vi "ContourPlot v2_no_I.vi"() -> ()   [LabVIEW 2024]
uses:
  <vilib>/Utility/file.llb/Read Delimited Spreadsheet (DBL).vi
  <vilib>/Analysis/NI_AALBase.lvlib
  <vilib>/gmath/NI_Gmath.lvlib
panel:
  out "Ready?":bool=TRUE
  in  "Auto x axis T":bool
  in  "Tab Control 2":enum32{"Contour", "Curve"}(tab)
  out "Intensity Graph":dbl[][](graph)
  out "XY Graph":cluster{"Y":dbl[], "Y":dbl[]}[](graph)=[{"Y"=[0.0, 0.1, 0.2, 0.3, 0.4, 0.5, 0.6, 0.7, 0.8, 0.9, 1.0, 1.1, 1.2, 1.3, 1.4, 1.5, 1.6, 1.7, 1.8, 1.9, 2.0, 2.1, 2.2, 2.3, 2.4, 2.5, 2.6, 2.7, 2.8, 2.9, 3.0, 3.1, 3.2, 3.3, 3.4, 3.5, 3.6, 3.7, 3.8, 3.9, 4.0, 4.1, 4.2, 4.3, 4.4, 4.5, 4.6, 4.7, 4.8, 4.9, 5.0, 4.9, 4.8, 4.7, 4.6, 4.5, 4.4, 4.3, 4.2, 4.1, 4.0, 3.9, 3.8, 3.7, 3.6, 3.5, 3.4, 3.3, 3.2, 3.1, 3.0, 2.9, 2.8, 2.7, 2.6, 2.5, 2.4, 2.3, 2.2, 2.1, 2.0, 1.9, 1.8, 1.7, 1.6, 1.5, 1.4, 1.3, 1.2, 1.1, 1.0, 0.9, 0.8, 0.7, 0.6, 0.5, 0.4, 0.3, 0.2, 0.1, 0.0, -0.1, -0.2, -0.3, -0.4, -0.5, -0.6, -0.7, -0.8, -0.9, -1.0, -1.1, -1.2, -1.3, -1.4, -1.5, -1.6, -1.7, -1.8, -1.9, -2.0, -2.1, -2.2, -2.3, -2.4, -2.5, -2.6, -2.7, -2.8, -2.9, -3.0, -3.1, -3.2, -3.3, -3.4, -3.5, -3.6, -3.7, -3.8, -3.9, -4.0, -4.1, -4.2, -4.3, -4.4, -4.5, -4.6, -4.7, -4.8, -4.9, -5.0, -4.9, -4.8, -4.7, -4.6, -4.5, -4.4, -4.3, -4.2, -4.1, -4.0, -3.9, -3.8, -3.7, -3.6, -3.5, -3.4, -3.3, -3.2, -3.1, -3.0, -2.9, -2.8, -2.7, -2.6, -2.5, -2.4, -2.3, -2.2, -2.1, -2.0, -1.9, -1.8, -1.7, -1.6, -1.5, -1.4, -1.3, -1.2, -1.1, -1.0, -0.9, -0.8, -0.7, -0.6, -0.5, -0.4, -0.3, -0.2, -0.1], "Y"=[-inf, -inf, -inf, -inf, -inf, -inf, -inf, -inf, -inf, -inf, -inf, -inf, -inf, -inf, -inf, -inf, -inf, -inf, 0.5607799884800001, 0.58669998848, 0.58669998848, 0.56749998848, 0.5578999884800001, 0.57805999616, 0.5502199961600001, 0.58285999424, -inf, -inf, -inf, -inf, -inf, 0.59917999424, 0.5905399884800001, 0.34573999616, 0.60301999616, 0.6529399884799999, 0.5290999884800001, 0.49549998848, 0.58669998848, 0.5953399884799999, 0.5876599884800001, 0.35149999616, 0.34478001152000004, 0.6097399884799999, 0.34765998848, 0.6250999884799999, 0.61933999424, 0.34478000576, 0.60493999616, 0.6030199884799999, 0.56653999424, 0.53389999424, 0.52717999616, 0.49645998848, 0.47725998848, 0.46477999711999995, 0.52429999424, 0.5358199884800001, 0.58957998848, 0.34478000576, 0.34765999424000005, 0.34478000576, -inf, -inf, 0.57805999424, 0.34478001152000004, -inf, -inf, 0.34573999616, -inf, -inf, -inf, -inf, -inf, -inf, -inf, -inf, -inf, -inf, -inf, -inf, -inf, -inf, -inf, -inf, -inf, -inf, -inf, -inf, -inf, -inf, -inf, -inf, -inf, -inf, -inf, -inf, -inf, -inf, -inf, -inf, -inf, -inf, -inf, -inf, -inf, -inf, -inf, -inf, -inf, -inf, -inf, -inf, -inf, -inf, -inf, -inf, -inf, -inf, -inf, -inf, -inf, 0.6519799884799999, -inf, -inf, 0.34765998848, 0.34669998848, -inf, 0.34478001152000004, 0.58957999424, 0.34573998848, 0.58957999616, 0.58957999424, 0.5550199884800001, 0.5886199884800001, 0.5617399884800001, 0.5905399884800001, 0.6519799884799999, 0.6202999942399999, 0.55309999424, 0.53005998848, 0.52045999424, 0.50509998848, 0.48109999423999994, 0.49741999616, 0.49453998847999997, 0.48301998848, 0.48301998848, 0.48109998847999996, 0.5310199884800001, 0.5905399884800001, 0.5905399884800001, 0.5262199884800001, 0.5646199884800001, 0.5905399884800001, 0.5751799884800001, 0.59629998848, 0.5818999980799999, 0.6164599884799999, 0.34478000576, -inf, -inf, -inf, -inf, -inf, 0.34573998848, -inf, -inf, 0.34478001152000004, -inf, 0.34478001152000004, -inf, -inf, -inf, -inf, -inf, -inf, -inf, -inf, -inf, -inf, -inf, -inf, -inf, -inf, -inf, -inf, -inf, -inf, -inf, -inf, -inf, 3.79790000576, 3.73550001152, -inf, -inf, -inf, -inf, -inf, -inf]}]
  in  "Voltage treshold":dbl=1.2e-05 format="%_3g"
  in  "Ignore points":i32=250
  in  "Tab Control":enum32{"Y cut ", "Y curve", "X cut"}(tab)=enum."Y curve"
  out "Y Cut":cluster{dbl[], "Intensity Graph":dbl[]}(graph)
  in  "intervals":i32=100
  out "Y Histogram":T1(graph)={"X Values"=[3.75038961, 3.75213283, 3.7538760499999997, 3.7556192699999995, 3.7573624899999993, 3.759105709999999, 3.760848929999999, 3.762592149999999, 3.7643353699999986, 3.7660785899999984, 3.7678218099999983, 3.769565029999998, 3.771308249999998, 3.7730514699999977, 3.7747946899999976, 3.7765379099999974, 3.778281129999997, 3.780024349999997, 3.781767569999997, 3.7835107899999967, 3.7852540099999965, 3.7869972299999963, 3.788740449999996, 3.790483669999996, 3.792226889999996, 3.7939701099999956, 3.7957133299999954, 3.7974565499999953, 3.799199769999995, 3.800942989999995, 3.8026862099999947, 3.8044294299999946, 3.8061726499999944, 3.807915869999994, 3.809659089999994, 3.811402309999994, 3.8131455299999937, 3.8148887499999935, 3.8166319699999933, 3.818375189999993, 3.820118409999993, 3.821861629999993, 3.8236048499999926, 3.8253480699999924, 3.8270912899999923, 3.828834509999992, 3.830577729999992, 3.8323209499999917, 3.8340641699999916, 3.8358073899999914, 3.837550609999991, 3.839293829999991, 3.841037049999991, 3.8427802699999907, 3.8445234899999905, 3.8462667099999903, 3.84800992999999, 3.84975314999999, 3.85149636999999, 3.8532395899999896, 3.8549828099999894, 3.8567260299999893, 3.858469249999989, 3.860212469999989, 3.8619556899999887, 3.8636989099999886, 3.8654421299999884, 3.867185349999988, 3.868928569999988, 3.870671789999988, 3.8724150099999877, 3.8741582299999875, 3.8759014499999873, 3.877644669999987, 3.879387889999987, 3.881131109999987, 3.8828743299999866, 3.8846175499999864, 3.8863607699999863, 3.888103989999986, 3.889847209999986, 3.8915904299999857, 3.8933336499999855, 3.8950768699999854, 3.896820089999985, 3.898563309999985, 3.900306529999985, 3.9020497499999847, 3.9037929699999845, 3.9055361899999843, 3.907279409999984, 3.909022629999984, 3.910765849999984, 3.9125090699999836, 3.9142522899999834, 3.9159955099999832, 3.917738729999983, 3.919481949999983, 3.9212251699999827, 3.9229683899999825], "Histogram: h(x)"=[1, 0, 0, 0, 0, 0, 0, 2, 0, 0, 0, 1, 0, 0, 1, 0, 1, 0, 0, 3, 2, 6, 5, 5, 4, 6, 5, 7, 5, 9, 11, 10, 7, 4, 13, 19, 20, 29, 21, 22, 20, 29, 41, 35, 44, 31, 43, 57, 50, 60, 68, 80, 88, 77, 95, 96, 111, 129, 153, 146, 164, 145, 201, 219, 230, 252, 254, 300, 343, 312, 361, 376, 335, 418, 424, 438, 448, 345, 399, 403, 331, 298, 293, 226, 209, 177, 126, 85, 86, 56, 28, 16, 15, 8, 2, 1, 1, 2, 0, 1]}
  in  "Histogram range":dbl=0.4
  out "X Cut":cluster{dbl[], "Intensity Graph":dbl[]}(graph)={[0.0, 0.1, 0.2, 0.30000000000000004, 0.4, 0.5, 0.6000000000000001, 0.7000000000000001, 0.8, 0.9, 1.0, 1.1, 1.2000000000000002, 1.3, 1.4000000000000001, 1.5, 1.6, 1.7000000000000002, 1.8, 1.9000000000000001, 2.0, 2.1, 2.2, 2.3000000000000003, 2.4000000000000004, 2.5, 2.6, 2.7, 2.8000000000000003, 2.9000000000000004, 3.0, 3.1, 3.2, 3.3000000000000003, 3.4000000000000004, 3.5, 3.6, 3.7, 3.8000000000000003, 3.9000000000000004, 4.0, 4.1000000000000005, 4.2, 4.3, 4.4, 4.5, 4.6000000000000005, 4.7, 4.800000000000001, 4.9, 5.0, 5.1000000000000005, 5.2, 5.300000000000001, 5.4, 5.5, 5.6000000000000005, 5.7, 5.800000000000001, 5.9, 6.0, 6.1000000000000005, 6.2, 6.300000000000001, 6.4, 6.5, 6.6000000000000005, 6.7, 6.800000000000001, 6.9, 7.0, 7.1000000000000005, 7.2, 7.300000000000001, 7.4, 7.5, 7.6000000000000005, 7.7, 7.800000000000001, 7.9, 8.0, 8.1, 8.200000000000001, 8.3, 8.4, 8.5, 8.6, 8.700000000000001, 8.8, 8.9, 9.0, 9.1, 9.200000000000001, 9.3, 9.4, 9.5, 9.600000000000001, 9.700000000000001, 9.8, 9.9, 10.0, 10.100000000000001, 10.200000000000001, 10.3, 10.4, 10.5, 10.600000000000001, 10.700000000000001, 10.8, 10.9, 11.0, 11.100000000000001, 11.200000000000001, 11.3, 11.4, 11.5, 11.600000000000001, 11.700000000000001, 11.8, 11.9, 12.0, 12.100000000000001, 12.200000000000001, 12.3, 12.4, 12.5, 12.600000000000001, 12.700000000000001, 12.8, 12.9, 13.0, 13.100000000000001, 13.200000000000001, 13.3, 13.4, 13.5, 13.600000000000001, 13.700000000000001, 13.8, 13.9, 14.0, 14.100000000000001, 14.200000000000001, 14.3, 14.4, 14.5, 14.600000000000001, 14.700000000000001, 14.8, 14.9, 15.0, 15.100000000000001, 15.200000000000001, 15.3, 15.4, 15.5, 15.600000000000001, 15.700000000000001, 15.8, 15.9, 16.0, 16.1, 16.2, 16.3, 16.400000000000002, 16.5, 16.6, 16.7, 16.8, 16.900000000000002, 17.0, 17.1, 17.2, 17.3, 17.400000000000002, 17.5, 17.6, 17.7, 17.8, 17.900000000000002, 18.0, 18.1, 18.2, 18.3, 18.400000000000002, 18.5, 18.6, 18.7, 18.8, 18.900000000000002, 19.0, 19.1, 19.200000000000003, 19.3, 19.400000000000002, 19.5, 19.6, 19.700000000000003, 19.8, 19.900000000000002], "Intensity Graph"=[0.0, 0.0, 0.0, 0.0, 0.0, 0.0, 4.0, 3.0, 0.0, 0.0, 0.0, 0.0, 0.0, 0.0, 0.0, 0.0, 0.0, 0.0, 0.0, 0.0, 0.0, 0.0, 0.0, 0.0, 0.0, 0.0, 0.0, 0.0, 0.0, 0.0, 0.0, 0.0, 0.0, 0.0, 0.0, 0.0, 0.0, 0.0, 0.0, 0.0, 0.0, 0.0, 0.0, 0.0, 0.0, 0.0, 0.0, 0.0, 0.0, 0.0, 0.0, 0.0, 0.0, 0.0, 0.0, 0.0, 0.0, 0.0, 0.0, 0.0, 0.0, 0.0, 0.0, 0.0, 0.0, 0.0, 0.0, 0.0, 0.0, 0.0, 0.0, 0.0, 0.0, 0.0, 0.0, 0.0, 0.0, 0.0, 0.0, 0.0, 0.0, 0.0, 0.0, 0.0, 0.0, 0.0, 0.0, 0.0, 0.0, 0.0, 0.0, 0.0, 0.0, 0.0, 0.0, 0.0, 0.0, 0.0, 0.0, 0.0, 0.0, 0.0, 0.0, 0.0, 0.0, 0.0, 114.0, 0.0, 0.0, 0.0, 0.0, 0.0, 0.0, 0.0, 0.0, 0.0, 0.0, 0.0, 0.0, 0.0, 0.0, 0.0, 0.0, 0.0, 0.0, 0.0, 0.0, 0.0, 0.0, 0.0, 0.0, 0.0, 0.0, 0.0, 0.0, 0.0, 0.0, 0.0, 0.0, 0.0, 0.0, 0.0, 0.0, 0.0, 0.0, 0.0, 0.0, 0.0, 0.0, 0.0, 0.0, 0.0, 0.0, 0.0, 0.0, 0.0, 0.0, 0.0, 0.0, 0.0, 0.0, 0.0, 0.0, 0.0, 0.0, 0.0, 0.0, 0.0, 0.0, 0.0, 0.0, 0.0, 0.0, 0.0, 0.0, 0.0, 0.0, 0.0, 0.0, 17.0, 0.0, 0.0, 0.0, 0.0, 0.0, 0.0, 0.0, 0.0, 0.0, 0.0, 0.0, 0.0, 0.0, 0.0, 0.0, 0.0, 0.0, 0.0, 0.0, 0.0]}
  in  "Normal T or Distribution F":bool
  in  "book number":i32=375
  in  "file path (dialog if empty)":path=path "C:/Users/gyue/Box/Guang Yue uiuc research box folder/data/Contour plot"
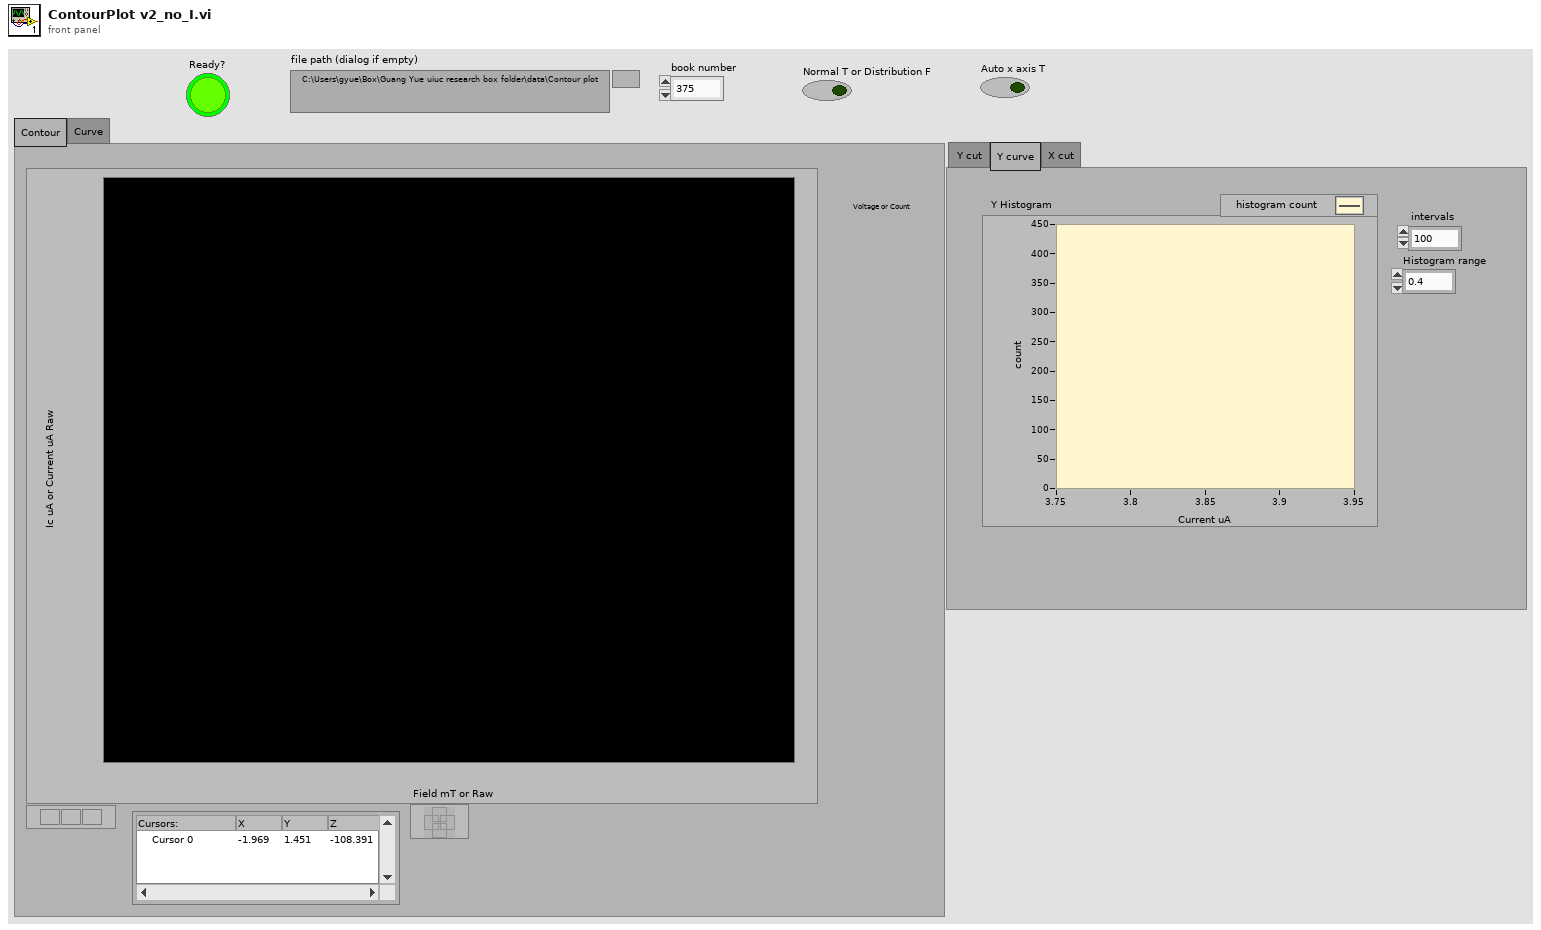
[diagram p1: front panel]
types:
  T1 = cluster{"X Values":dbl[], "Histogram: h(x)":i32[]}
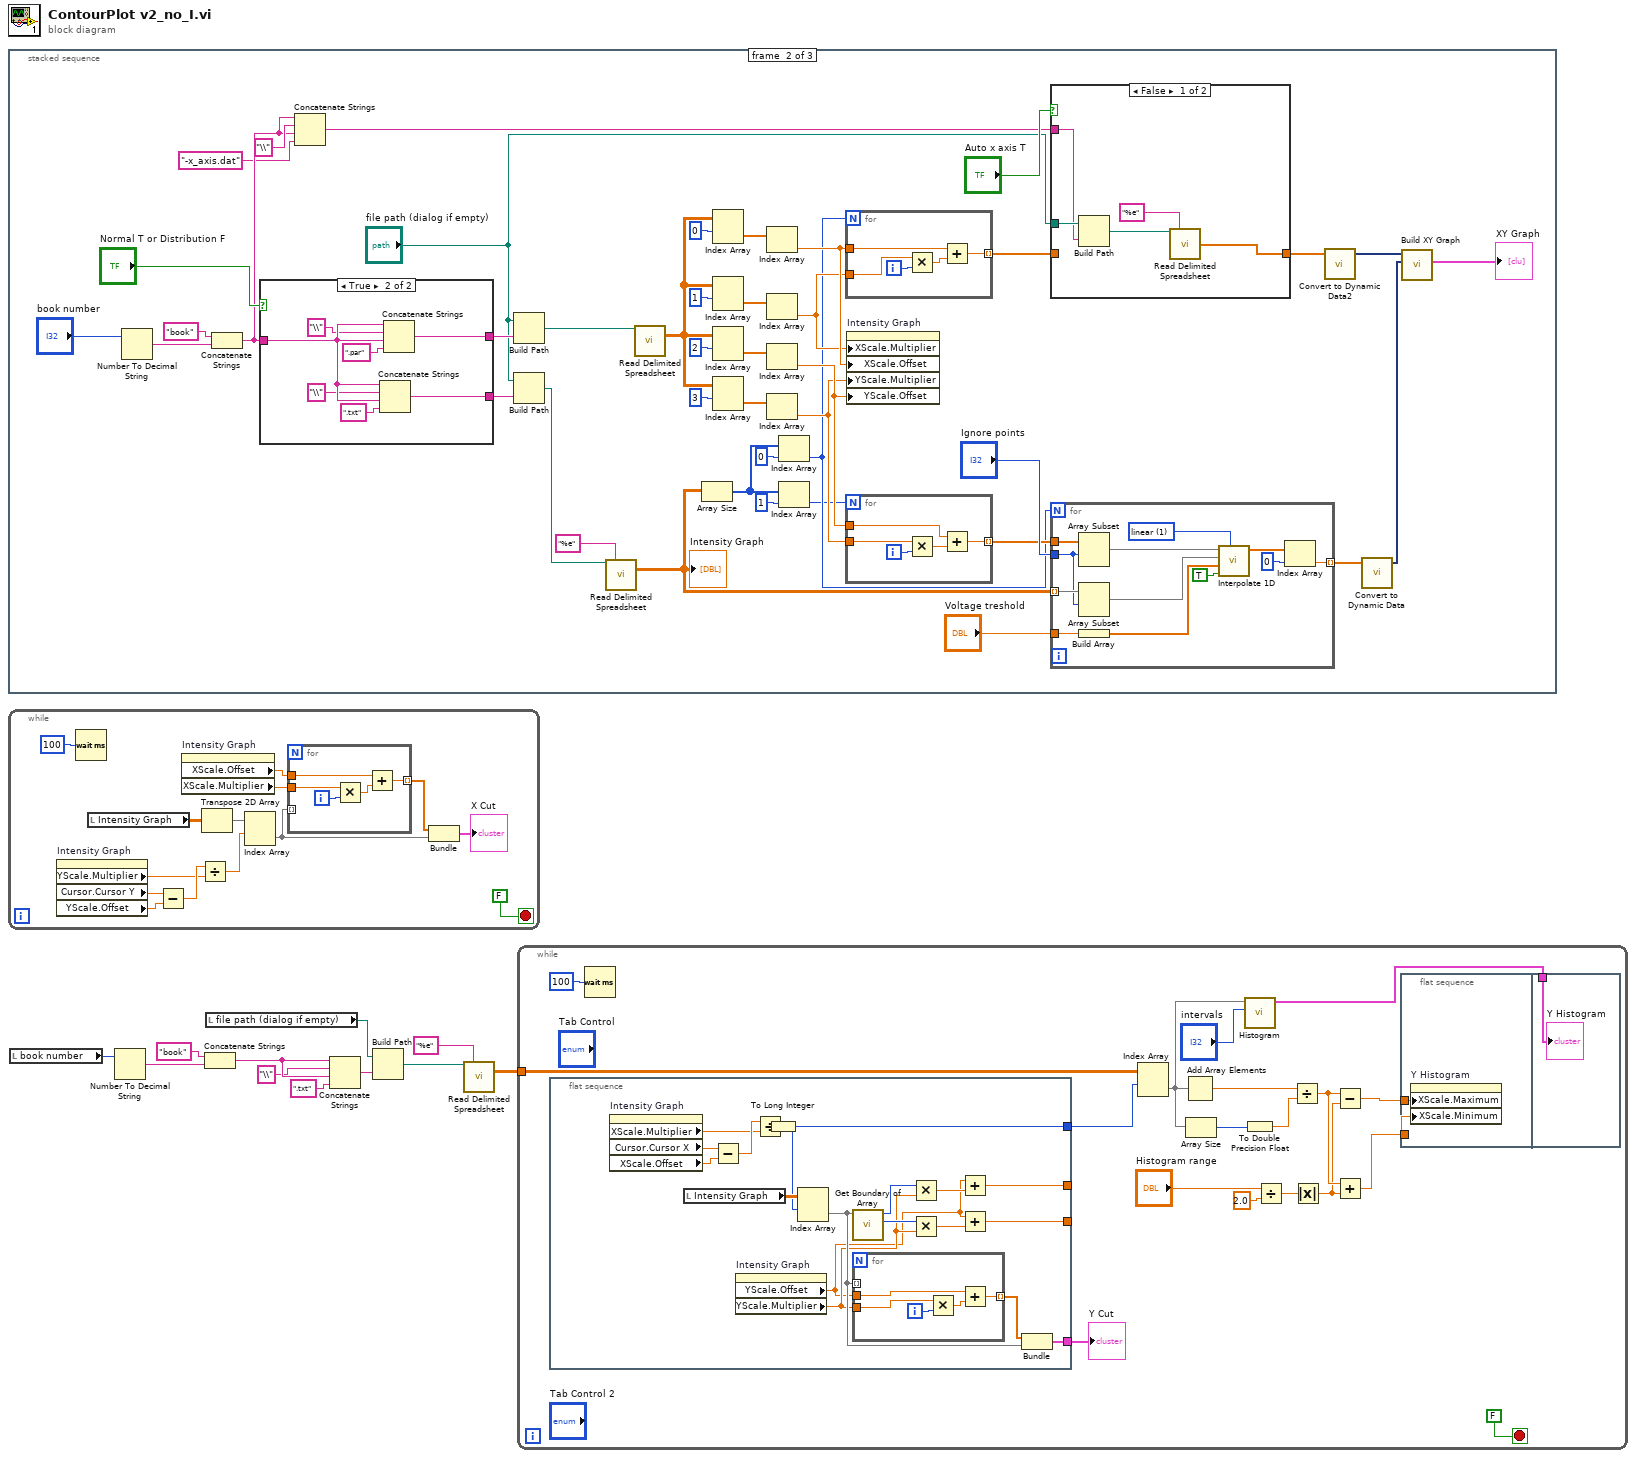
[diagram p0: block diagram]
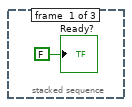
[diagram p2: hidden frame]
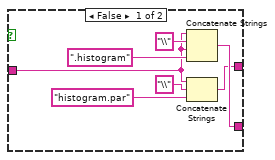
[diagram p4: hidden frame]
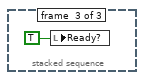
[diagram p5: hidden frame]
diagram:
  n1 = stacked-sequence {
    frame #0 {
      "Ready?" <- FALSE ("Ready?")
    }
    frame #1 {
      n2 = Number To Decimal String(number="book number") -> (decimal integer string=w51:string)  [unwired: 1 in]
      n3 = Concatenate Strings("book" ("string"), w51) -> (w20:string)
      n4 = case shown="True" "Normal T or Distribution F" {
        tunnel: [w86 w97] -> w53
        tunnel: w20 -> [w85 w95]
        tunnel: [w87 w93] -> w52
        frame False {
          n5 = Concatenate Strings(w85, "\\" ("string"), w85, ".histogram" ("string")) -> (w87:string)
          n6 = Concatenate Strings(w85, "\\" ("string"), "histogram.par" ("string")) -> (w86:string)
        }
        frame True {
          n7 = Concatenate Strings(w95, "\\" ("string"), w95, ".txt" ("string")) -> (w93:string)
          n8 = Concatenate Strings(w95, "\\" ("string"), w95, ".par" ("string")) -> (w97:string)
        }
      }
      n9 = Concatenate Strings(w20, "\\" ("string"), w20, "-x_axis.dat" ("string")) -> (w17:string)
      n10 = Build Path(base path="file path (dialog if empty)", name or relative path=w53) -> (appended path=w54:path)
      n11 = Build Path(base path="file path (dialog if empty)", name or relative path=w52) -> (appended path=w55:path)
      n12 = call-poly <vilib>:"Read Delimited Spreadsheet.vi"("file path (dialog if empty)"=w55, "format (%.3f)"="%e") -> ("all rows"=w37:dbl[][])  [unwired: 8 in, 5 out]
      "Intensity Graph" <- w37
      n13 = call-poly <vilib>:"Read Delimited Spreadsheet.vi"("file path (dialog if empty)"=w54) -> ("all rows"=w47:dbl[][])  [unwired: 9 in, 5 out]
      n14 = Array Size(array=w37) -> (size(s)=w16:i32[])
      n15 = Index Array(array=w47, index (row)=0) -> (element=w44:dbl[])  [unwired: 1 in]
      n16 = Index Array(array=w47, index (row)=1) -> (element=w43:dbl[])  [unwired: 1 in]
      n17 = Index Array(array=w47, index (row)=2) -> (element=w42:dbl[])  [unwired: 1 in]
      n18 = Index Array(array=w47, index (row)=3) -> (element=w41:dbl[])  [unwired: 1 in]
      n19 = Index Array(array=w44) -> (element=w34:dbl)  [unwired: 1 in]
      n20 = Index Array(array=w43) -> (element=w33:dbl)  [unwired: 1 in]
      n21 = Index Array(array=w42) -> (element=w36:dbl)  [unwired: 1 in]
      n22 = Index Array(array=w41) -> (element=w35:dbl)  [unwired: 1 in]
      n23 = Index Array(array=w16, index=0) -> (element=w14:i32)
      n24 = Index Array(array=w16, index=1) -> (element=w13:i32)
      n25 = for {
        N: w14 -> [_]
        tunnel: w34 -> [w66]
        tunnel: w33 -> [w64]
        tunnel: [w62] -> w23 mode=indexing
        i -> [w65]
        n26 = Multiply(x=w64, y=w65) -> (x*y=w63:dbl)
        n27 = Add(x=w66, y=w63) -> (x+y=w62:dbl)
      }
      n28 = for {
        N: w13 -> [_]
        tunnel: w36 -> [w71]
        tunnel: w35 -> [w69]
        tunnel: [w67] -> w25 mode=indexing
        i -> [w70]
        n29 = Multiply(x=w69, y=w70) -> (x*y=w68:dbl)
        n30 = Add(x=w71, y=w68) -> (x+y=w67:dbl)
      }
      n31 = property on="Intensity Graph" class="IntGraph (strict)"("XScale.Multiplier"=w33, "XScale.Offset"=w34, "YScale.Multiplier"=w35, "YScale.Offset"=w36) -> ()  [unwired: 2 in, 2 out]
      n32 = case shown="False" "Auto x axis T" {
        tunnel: w23 -> [_ w61]
        tunnel: [w56 w61] -> w22
        tunnel: "file path (dialog if empty)" -> [w60 _]
        tunnel: w17 -> [w59 _]
        frame False {
          n33 = Build Path(base path=w60, name or relative path=w59) -> (appended path=w58:path)
          n34 = call-poly <vilib>:"Read Delimited Spreadsheet.vi"("file path (dialog if empty)"=w58, "format (%.3f)"="%e") -> ("first row"=w56:dbl[])  [unwired: 8 in, 5 out]
        }
        frame True {
        }
      }
      n35 = for {
        N: w14 -> [_]
        tunnel: w37 -> [w76] mode=indexing
        tunnel: w25 -> [w77]
        tunnel: [w78] -> w31 mode=indexing
        tunnel: "Ignore points" -> [w72]
        tunnel: "Voltage treshold" -> [w73]
        w82 = 1 items=["nearest", "linear", "spline", "cubic Hermite", "Lagrange"] ("method")
        n36 = Array Subset(array=w77, index=w72) -> (w74:dbl[])  [unwired: 1 in]
        n37 = Array Subset(array=w76, index=w72) -> (w75:dbl[])  [unwired: 1 in]
        n38 = Build Array(w73) -> (w81:dbl[])
        n39 = call <vilib>:"Interpolate 1D.vi"("method"=w82, "X is monotonic"=TRUE, "xi"=w81, "X"=w75, "Y"=w74) -> ("yi"=w80:dbl[])  [unwired: 4 in, 2 out]
        n40 = Index Array(array=w80, index=0) -> (element=w78:dbl)
      }
      n41 = call "Convert to Dynamic Data2"("Array"=w22) -> ("Dynamic Data Type"=w29:dynamicdata)  [unwired: 3 in]
      n42 = call "Convert to Dynamic Data"("Array"=w31) -> ("Dynamic Data Type"=w30:dynamicdata)  [unwired: 3 in]
      n43 = call "Build XY Graph"("Y Input"=w30, "X Input"=w29) -> ("XY Graph"=→"XY Graph":cluster{"X":dbl[], "Y":dbl[]}[])  [unwired: 8 in, 1 out]
    }
    frame #2 {
      n44 = local write "Ready?"(TRUE ("Ready?")) -> ()
    }
  }
  n45 = while {
    stop <- FALSE stop-if-true
    n46 = property on="Intensity Graph" class="IntGraph (strict)"() -> ("YScale.Multiplier"=w107:dbl, "Cursor.Cursor Y"=w106:dbl, "YScale.Offset"=w105:dbl)  [unwired: 2 in, 2 out]
    n47 = Wait (ms)(milliseconds to wait=u32 100) -> ()  [unwired: 1 out]
    n48 = local read "Intensity Graph"() -> (w102:dbl[][])
    n49 = Subtract(x=w106, y=w105) -> (x-y=w112:dbl)
    n50 = property on="Intensity Graph" class="IntGraph (strict)"() -> ("XScale.Offset"=w108:dbl, "XScale.Multiplier"=w109:dbl)  [unwired: 2 in, 2 out]
    n51 = Divide(x=w112, y=w107) -> (x/y=w111:dbl)
    n52 = Transpose 2D Array(2D array=w102) -> (transposed array=w101:dbl[][])
    n53 = Index Array(array=w101, index (row)=w111) -> (element=w103:dbl[])  [unwired: 1 in]
    n54 = for {
      tunnel: w109 -> [w116]
      tunnel: w108 -> [w114]
      tunnel: [w113] -> w110 mode=indexing
      tunnel: w103 -> [_] mode=indexing
      i -> [w117]
      n55 = Multiply(x=w116, y=w117) -> (x*y=w115:dbl)
      n56 = Add(x=w114, y=w115) -> (x+y=w113:dbl)
    }
    n57 = Bundle(w110, w103) -> (→"X Cut":cluster{dbl[], dbl[]})  [unwired: 1 in]
  }
  n58 = local read "book number"() -> (w6:i32)
  n59 = Number To Decimal String(number=w6) -> (decimal integer string=w5:string)  [unwired: 1 in]
  n60 = Concatenate Strings("book" ("string"), w5) -> (w7:string)
  n61 = local read "file path (dialog if empty)"() -> (w8:path)
  n62 = Concatenate Strings(w7, "\\" ("string"), w7, ".txt" ("string")) -> (w9:string)
  n63 = Build Path(base path=w8, name or relative path=w9) -> (appended path=w10:path)
  n64 = call-poly <vilib>:"Read Delimited Spreadsheet.vi"("file path (dialog if empty)"=w10, "format (%.3f)"="%e") -> ("all rows"=w11:dbl[][])  [unwired: 8 in, 5 out]
  n65 = while {
    tunnel: w11 -> [w131]
    stop <- FALSE stop-if-true
    n66 = flat-sequence {
      tunnel: [w151] -> w135
      tunnel: [w143] -> _
      tunnel: [w142] -> _
      tunnel: [w139] -> w132
      frame #0 {
        n67 = property on="Intensity Graph" class="IntGraph (strict)"() -> ("XScale.Multiplier"=w154:dbl, "Cursor.Cursor X"=w153:dbl, "XScale.Offset"=w152:dbl)  [unwired: 2 in, 2 out]
        n68 = local read "Intensity Graph"() -> (w155:dbl[][])
        n69 = Subtract(x=w153, y=w152) -> (x-y=w156:dbl)
        n70 = property on="Intensity Graph" class="IntGraph (strict)"() -> ("YScale.Offset"=w144:dbl, "YScale.Multiplier"=w145:dbl)  [unwired: 2 in, 2 out]
        n71 = Divide(x=w156, y=w154) -> (x/y=w141:dbl)
        n72 = To Long Integer(number=w141) -> (32bit integer=w139:i32)
        n73 = Index Array(array=w155, index (row)=w139) -> (element=w150:dbl[])  [unwired: 1 in]
        n74 = call "Get Boundary of Array.vi"("Array"=w150) -> ("Up"=w146:i32, "Down"=w149:i32)  [unwired: 9 in]
        n75 = for {
          tunnel: w145 -> [w160]
          tunnel: w144 -> [w158]
          tunnel: [w157] -> w140 mode=indexing
          tunnel: w150 -> [_] mode=indexing
          i -> [w161]
          n76 = Multiply(x=w160, y=w161) -> (x*y=w159:dbl)
          n77 = Add(x=w158, y=w159) -> (x+y=w157:dbl)
        }
        n78 = Multiply(x=w149, y=w145) -> (x*y=w148:dbl)
        n79 = Multiply(x=w146, y=w145) -> (x*y=w147:dbl)
        n80 = Add(x=w144, y=w148) -> (x+y=w143:dbl)
        n81 = Add(x=w144, y=w147) -> (x+y=w142:dbl)
        n82 = Bundle(w140, "Intensity Graph"=w150) -> (w151:cluster{dbl[], "Intensity Graph":dbl[]})  [unwired: 1 in]
      }
    }
    n83 = Wait (ms)(milliseconds to wait=u32 100) -> ()  [unwired: 1 out]
    n84 = Index Array(array=w131, index (row)=w132) -> (element=w121:dbl[])  [unwired: 1 in]
    n85 = Add Array Elements(numeric array=w121) -> (sum=w127:dbl)
    n86 = Array Size(array=w121) -> (size(s)=w126:i32)
    n87 = call <vilib>:"Histogram.vi"("intervals"="intervals", "X"=w121) -> ("Histogram Graph"=w118:T1)  [unwired: 6 in, 3 out]
    n88 = To Double Precision Float(number=w126) -> (double precision float=w125:dbl)
    n89 = Divide(x="Histogram range", y=2.0) -> (x/y=w124:dbl)
    n90 = Divide(x=w127, y=w125) -> (x/y=w123:dbl)
    n91 = Absolute Value(x=w124) -> (abs(x)=w122:dbl)
    n92 = Subtract(x=w123, y=w122) -> (x-y=w120:dbl)
    n93 = Add(x=w123, y=w122) -> (x+y=w119:dbl)
    n94 = flat-sequence {
      tunnel: w120 -> [w137]
      tunnel: w119 -> [w136]
      tunnel: w118 -> [w138]
      frame #0 {
        n95 = property on="Y Histogram" class="XYGraph (strict)"("XScale.Maximum"=w137, "XScale.Minimum"=w136) -> ()  [unwired: 2 in, 2 out]
      }
      frame #1 {
        "Y Histogram" <- w138
      }
    }
    "Y Cut" <- w135
  }
